vi "Main.vi"() -> ()   [LabVIEW 2018]
panel:
  out "Temp Dif  Down":dbl[unit](slide) scale=15.0..70.0
  out "Temp Dif  Up":dbl[unit](slide) scale=15.0..70.0
  out "Target Flow Evaporation Water":dbl[unit](slide)
  out "Temp Dif Down":dbl[unit]
  out "Temp Dif  Up":dbl[unit]
  out "Target Flow Evaporation Water":dbl[unit]
  out "Comp":bool
  in  "The Data are Stable\nPlease Save them!":bool
  in  "element 12":string
  in  "element 13":string
  in  "element 14":string
  in  "FileName":string="data"
  out "Temp Eva Water IN":dbl[unit]
  out "Run Program":bool
  out "Voltage Level FlowMeter Air ZeroFlow":dbl
  out "Voltage Level FlowMeter.Pre.EVA Ziro Flow Water":dbl
  out "Voltage Level FlowMeter.EVA ZiroFlow Water":dbl
  out "Humidity 3rd":dbl
  out "Humidity Evaporator IN":dbl
  out "Humidity Evaporator OUT":dbl
  out "Temp 3rd Air":dbl[unit]
  out "Temp Evaporator Air IN":dbl[unit]
  out "Temp Evaporator Air OUT":dbl[unit]
  out "Voltage Level Flowmeter Air":dbl
  out "Voltage Level Flowmeter.Pre Eva Water":dbl
  out "Voltage Level Flowmeter.EVA Water":dbl
  out "Temp water  Series 2":dbl[unit]
  out "Temp Pre Eva  Water OUT":dbl[unit]
  out "Temp Pre Eva water IN":dbl[unit]
  out "Temp Evaporator Water IN":dbl[unit]
  out "Temp Evaporator Water  Out":dbl[unit]
  in  "Calibration":bool
  out "SHT/H":dbl[](array[numeric])
  out "SHT/T":dbl[unit][](array[numeric])
  out "EEP":dbl[](array[numeric])
  out "MPX":dbl[](array[numeric])
  out "DS18b20":dbl[unit][](array[numeric])
  out "Flow Evaporation Water Detected by sensor":dbl[unit](slide)
  out "Flow Evaporation Water Detected by sensor":dbl[unit]
  out "S1 is greater Than S2\nThat is Wrong":bool
  out "T_WD":dbl[unit]
  out "Temp Eva Water Out":dbl[unit](slide) scale=15.0..70.0
  out "Temp Eva Air OUT":dbl[unit](slide) scale=15.0..70.0
  out "LMTD":dbl[unit](knob) scale=0.0..5.0
  out "LMTD":dbl[unit]
  out "Pre Evaporation Water Flow Detected by sensor":dbl[unit]
  out "Pre Evaporation Water Flow Detected by sensor":dbl[unit](slide)
  out "Temp Eva Air IN":dbl[unit](slide) scale=15.0..70.0
  out "Humidity Evaporator Air Input":dbl(knob) scale=30.0..100.0
  out "Temp Eva Water IN":dbl[unit](slide) scale=15.0..70.0
  out "MFRHA\nMass Flow Rate of Humid Air \nof Input(Kg/s)":dbl[unit]
  out "Added Vapor (kg/s)":dbl[unit]
  out "Total Transferd Energy of Air":dbl[unit]
  out "Total Transferd Energy of Air":dbl[unit](knob)
  out "Mass Flow Rate of Coil Water":dbl[unit]
  out "Mass Flow Rate of Coil Water":dbl[unit](slide)
  out "Temp Eva Air IN":dbl[unit]
  out "Humidity Evaporator Air Input":dbl
  in  "Gas Presure":dbl[unit]=80000.0 min=80000.0 max=120000.0
  out "Humidity Evaporator Air OUT\nRH Heat Exchanger Quality":dbl
  out "Humidity Evaporator Air OUT\nRH Heat Exchanger Quality":dbl(knob) scale=30.0..100.0
  out "Temp Eva Air OUT":dbl[unit]
  in  "stop":bool
  in  "Run Program":bool
  out "PortName":string
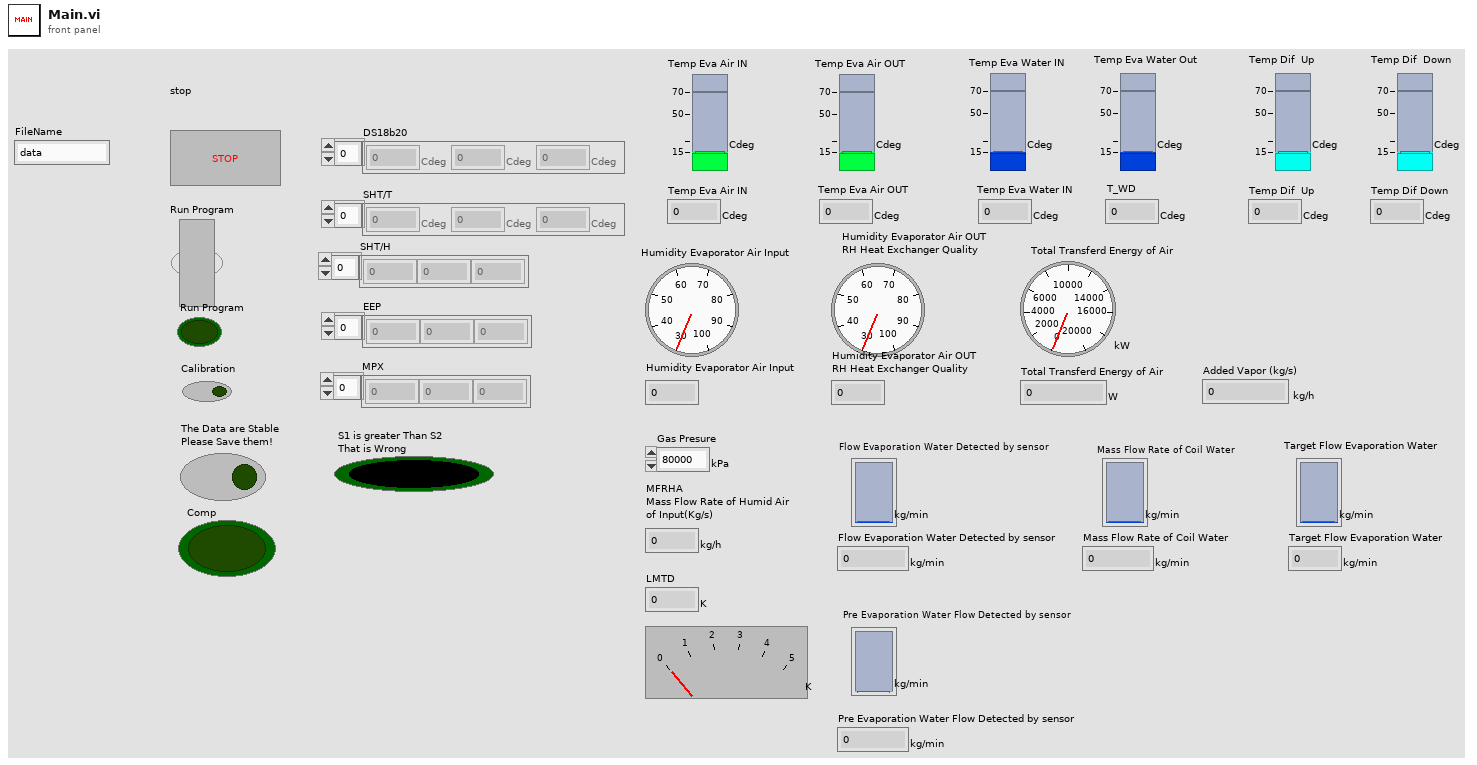
[diagram p1: front panel]
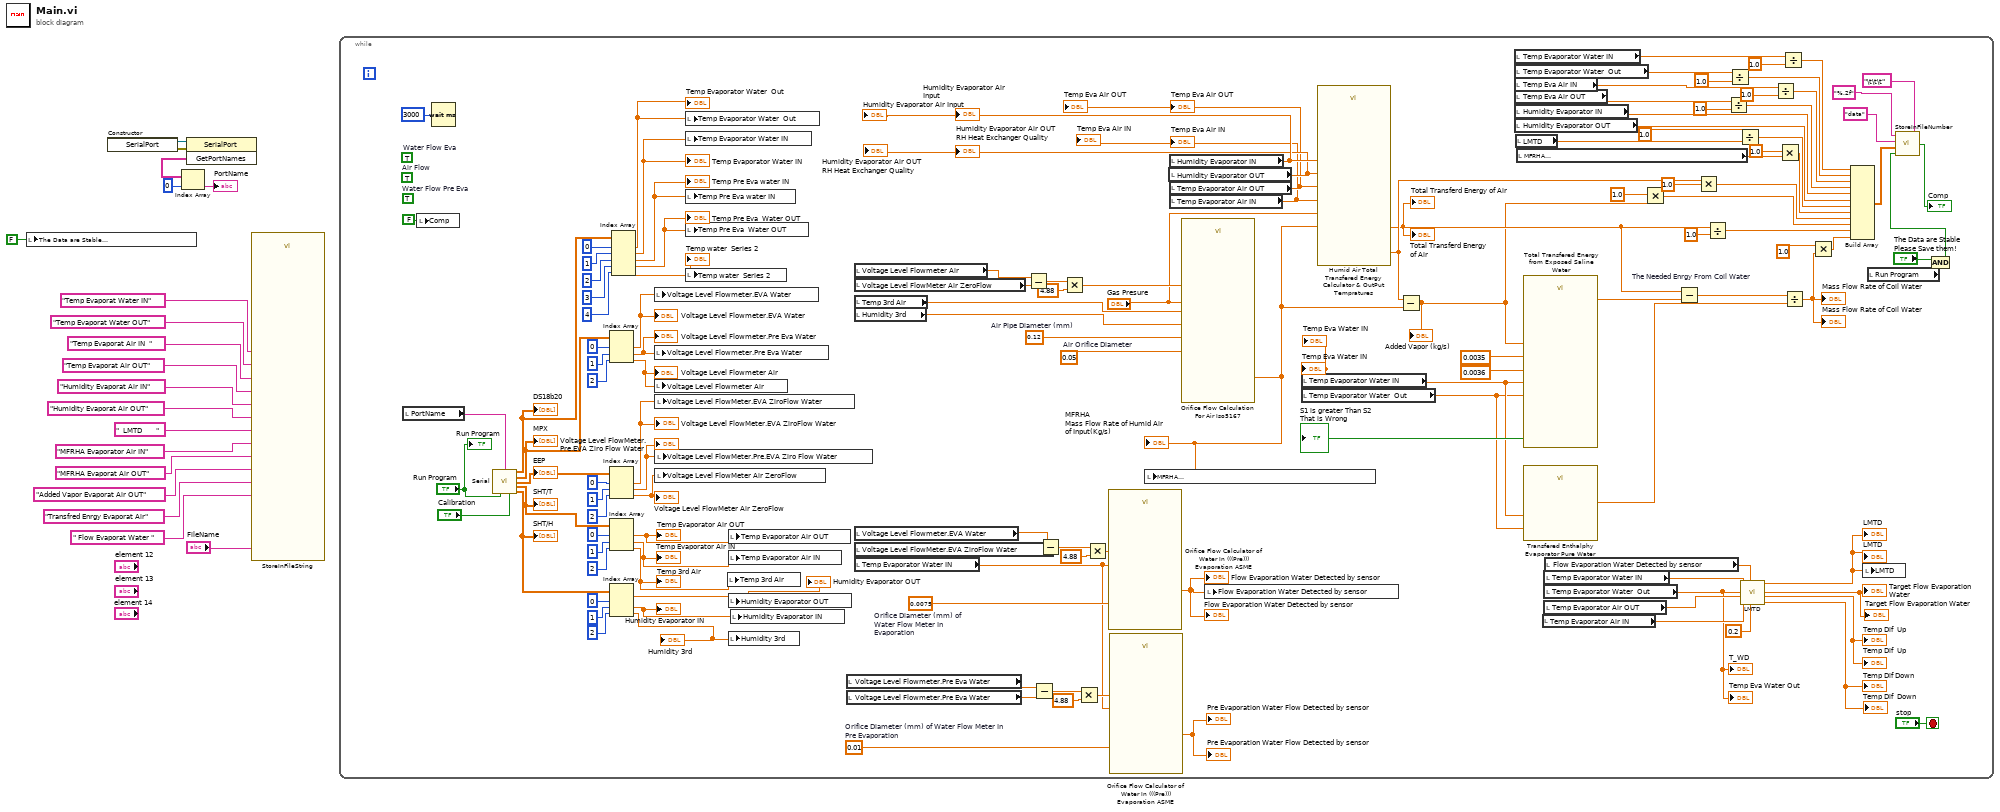
[diagram p0: block diagram]
diagram:
  n1 = local write "The Data are Stable\nPlease Save them!"(FALSE ("The Data are Stable\nPlease Save them!")) -> ()
  n2 = constructor class="SerialPort"() -> (reference out=w17:refnum<k24>, error out=w18:errorcluster)  [unwired: 3 in, 1 out]
  n3 = invoke class="SerialPort" method="GetPortNames"(reference=w17, error in=w18) -> ("GetPortNames"=w16:string[])  [unwired: 1 in, 2 out]
  n4 = Index Array(array=w16, index=0) -> (element=→"PortName":string)
  n5 = call "StoreInFileString.vi"("element0"="Temp Evaporat Water IN", "element 5"="Humidity Evaporat Air OUT", "element 6"="  LMTD       ", "element 7"="MFRHA Evaporator Air IN", "element 8"="MFRHA Evaporat Air OUT" ("element 9"), "element1"="Temp Evaporat Water OUT", "element 9"="Added Vapor Evaporat Air OUT" ("element 8"), "element 2"="Temp Evaporat Air IN  ", "element 10"="Transfred Enrgy Evaporat Air" ("element 11"), "element 3"="Temp Evaporat Air OUT", "element 11"=" Flow Evaporat Water " ("element 10"), "element 4"="Humidity Evaporat Air IN", "FileName"="FileName") -> ()  [unwired: 3 in]
  n6 = while {
    stop <- "stop" stop-if-true
    w138 = dbl[unit] 0.0075  # Orifice Diameter (mm) of Water Flow Meter In Evaporation
    w150 = dbl[unit] 0.12  # Air Pipe Diameter (mm)
    w97 = dbl[unit] 0.05  # Air Orifice Diameter
    w142 = dbl[unit] 0.01  # Orifice Diameter (mm) of Water Flow Meter In Pre Evaporation
    (unwired) TRUE  # Water Flow Eva
    (unwired) TRUE  # Water Flow Pre Eva
    (unwired) TRUE  # Air Flow
    n7 = local read "PortName"() -> (w79:string)
    n8 = local write "Comp"(FALSE ("Comp")) -> ()
    n9 = Wait (ms)(milliseconds to wait=u32 3000) -> ()  [unwired: 1 out]
    n10 = call "Serial.vi"("PortName"=w79, "Run"="Run Program", "Calibration"="Calibration") -> ("DS18b20"=w136:dbl[unit][], "MPX"=w130:dbl[], "EEP"=w115:dbl[], "SHT/H"=w126:dbl[unit][], "SHT/T"=w116:dbl[])  [unwired: 3 in, 5 out]
    "DS18b20" <- w136
    "MPX" <- w130
    "EEP" <- w115
    "SHT/T" <- w126
    "SHT/H" <- w116
    n11 = Index Array(array=w130, index #1=0 ("index"), index #2=1 ("index"), index #3=2 ("index")) -> (element #1=w111:dbl, element #2=w110:dbl, element #3=w100:dbl)
    "Voltage Level Flowmeter.EVA Water" <- w111
    "Voltage Level Flowmeter.Pre Eva Water" <- w110
    "Voltage Level Flowmeter Air" <- w100
    n12 = Index Array(array=w115, index #1=0 ("index"), index #2=1 ("index"), index #3=2 ("index")) -> (element #1=w109:dbl, element #2=w108:dbl, element #3=w107:dbl)
    "Voltage Level FlowMeter.EVA ZiroFlow Water" <- w109
    "Voltage Level FlowMeter.Pre.EVA Ziro Flow Water" <- w108
    "Voltage Level FlowMeter Air ZeroFlow" <- w107
    n13 = Index Array(array=w126, index #1=0 ("index"), index #2=1 ("index"), index #3=2 ("index")) -> (element #1=w105:dbl[unit], element #2=w106:dbl[unit], element #3=w104:dbl[unit])
    "Temp Evaporator Air OUT" <- w105
    "Temp Evaporator Air IN" <- w106
    "Temp 3rd Air" <- w104
    n14 = Index Array(array=w116, index #1=0 ("index"), index #2=1 ("index"), index #3=2 ("index")) -> (element #1=w102:dbl, element #2=w85:dbl, element #3=w103:dbl)
    "Humidity Evaporator OUT" <- w102
    "Humidity Evaporator IN" <- w85
    "Humidity 3rd" <- w103
    n15 = Index Array(array=w136, index #1=0 ("index"), index #2=1 ("index"), index #3=2 ("index"), index #4=3 ("index"), index #5=4 ("index")) -> (element #1=w68:dbl[unit], element #2=w91:dbl[unit], element #3=w119:dbl[unit], element #4=w118:dbl[unit], element #5=w117:dbl[unit])
    "Temp Evaporator Water  Out" <- w68
    "Temp Evaporator Water IN" <- w91
    "Temp Pre Eva water IN" <- w119
    "Temp Pre Eva  Water OUT" <- w118
    "Temp water  Series 2" <- w117
    n16 = local write "Voltage Level Flowmeter.EVA Water"(w111) -> ()
    n17 = local write "Voltage Level Flowmeter.Pre Eva Water"(w110) -> ()
    n18 = local write "Voltage Level Flowmeter Air"(w100) -> ()
    n19 = local write "Voltage Level FlowMeter.EVA ZiroFlow Water"(w109) -> ()
    n20 = local write "Voltage Level FlowMeter.Pre.EVA Ziro Flow Water"(w108) -> ()
    n21 = local write "Voltage Level FlowMeter Air ZeroFlow"(w107) -> ()
    n22 = local write "Temp Evaporator Water  Out"(w68) -> ()
    n23 = local write "Temp Evaporator Water IN"(w91) -> ()
    n24 = local write "Temp Pre Eva water IN"(w119) -> ()
    n25 = local write "Temp Pre Eva  Water OUT"(w118) -> ()
    n26 = local write "Temp water  Series 2"(w117) -> ()
    n27 = local write "Temp 3rd Air"(w104) -> ()
    n28 = local write "Temp Evaporator Air OUT"(w105) -> ()
    n29 = local write "Temp Evaporator Air IN"(w106) -> ()
    n30 = local write "Humidity Evaporator OUT"(w102) -> ()
    n31 = local write "Humidity 3rd"(w103) -> ()
    n32 = local write "Humidity Evaporator IN"(w85) -> ()
    n33 = local read "Voltage Level Flowmeter.Pre Eva Water"() -> (w96:dbl)
    n34 = local read "Voltage Level Flowmeter.Pre Eva Water"() -> (w95:dbl)
    n35 = local read "Voltage Level Flowmeter Air"() -> (w101:dbl)
    n36 = local read "Voltage Level FlowMeter Air ZeroFlow"() -> (w99:dbl)
    n37 = local read "Temp 3rd Air"() -> (w86:dbl[unit])
    n38 = local read "Humidity 3rd"() -> (w87:dbl)
    n39 = local read "Voltage Level Flowmeter.EVA Water"() -> (w94:dbl)
    n40 = local read "Voltage Level FlowMeter.EVA ZiroFlow Water"() -> (w93:dbl)
    n41 = local read "Temp Evaporator Water IN"() -> (w92:dbl[unit])
    n42 = Subtract(x=w101, y=w99) -> (x-y=w147:dbl)
    n43 = Subtract(x=w96, y=w95) -> (x-y=w144:dbl)
    n44 = Subtract(x=w94, y=w93) -> (x-y=w140:dbl)
    n45 = Multiply(x=w147, y=dbl[unit] 4.88) -> (x*y=w151:dbl[unit])
    n46 = Multiply(x=w144, y=dbl[unit] 4.88) -> (x*y=w143:dbl[unit])
    n47 = Multiply(x=w140, y=dbl[unit] 4.88) -> (x*y=w139:dbl[unit])
    n48 = call "Orifice Flow Calculator of Water In (((Pre))) Evaporation ASME.vi"("Water Temperature"=w92, "Delta P\n(Presure Made By Orifice)"=w139, "Orifice Diameter"=w138) -> ("Mass Flow (Orifice) (Kg/min)"=w33:dbl[unit])  [unwired: 1 in, 2 out]
    "Flow Evaporation Water Detected by sensor" <- w33
    "Flow Evaporation Water Detected by sensor" <- w33
    n49 = call "Orifice Flow Calculator of Water In (((Pre))) Evaporation ASME.vi"("Water Temperature"=w92, "Delta P\n(Presure Made By Orifice)"=w143, "Orifice Diameter"=w142) -> ("Mass Flow (Orifice) (Kg/min)"=→"Pre Evaporation Water Flow Detected by sensor" →"Pre Evaporation Water Flow Detected by sensor":dbl[unit])  [unwired: 1 in, 2 out]
    n50 = local read "Humidity Evaporator OUT"() -> (w83:dbl)
    "Humidity Evaporator Air OUT\nRH Heat Exchanger Quality" <- w83
    "Humidity Evaporator Air OUT\nRH Heat Exchanger Quality" <- w83
    n51 = local read "Humidity Evaporator IN"() -> (w84:dbl)
    "Humidity Evaporator Air Input" <- w84
    "Humidity Evaporator Air Input" <- w84
    n52 = local read "Temp Evaporator Air OUT"() -> (w81:dbl[unit])
    "Temp Eva Air OUT" <- w81
    "Temp Eva Air OUT" <- w81
    n53 = local read "Temp Evaporator Air IN"() -> (w80:dbl[unit])
    "Temp Eva Air IN" <- w80
    "Temp Eva Air IN" <- w80
    n54 = call "Orifice Flow Calculation For Air Iso5167.vi"("RH"=w87, "Orifice Diameter"=w97, "Gas Temperature"=w86, "P1\n(Presure After Fan &\n before Orifice)"="Gas Presure", "Pipe Diameter (mm)"=w150, "Delta P\n(Presure Made By Orifice)"=w151) -> ("Mass Flow (Orifice) (Kg/h)"=w47:dbl[unit])  [unwired: 2 out]
    "MFRHA\nMass Flow Rate of Humid Air \nof Input(Kg/s)" <- w47
    n55 = local write "MFRHA\nMass Flow Rate of Humid Air \nof Input(Kg/s)"(w47) -> ()
    n56 = local write "Flow Evaporation Water Detected by sensor"(w33) -> ()
    n57 = local read "Temp Evaporator Water IN"() -> (w22:dbl[unit])
    "Temp Eva Water IN" <- w22
    "Temp Eva Water IN" <- w22
    n58 = local read "Temp Evaporator Water  Out"() -> (w21:dbl[unit])
    n59 = call "Humid Air Total Transfered Energy Calculator & OutPut Tempratures.vi"("MFRHA\nMass Flow Rate of Humid Air (Kg/s)"=w47, "Gas Presure"="Gas Presure", "T_AU"=w81, "Tceg"=w80, "RH Heat Exchanger Quality"=w83, "RH"=w84) -> ("Mass Flow Rate of Humid Air of Out Put"=w66:dbl[unit], "ToTal Transferd Energy of Air"=w64:dbl[unit])
    "Total Transferd Energy of Air" <- w64
    "Total Transferd Energy of Air" <- w64
    n60 = Subtract(x=w66, y=w47) -> (x-y=w26:dbl[unit])
    "Added Vapor (kg/s)" <- w26
    n61 = local read "Temp Evaporator Water IN"() -> (w76:dbl[unit])
    n62 = local read "Temp Evaporator Water  Out"() -> (w71:dbl[unit])
    n63 = local read "Temp Eva Air IN"() -> (w70:dbl[unit])
    n64 = local read "Temp Eva Air OUT"() -> (w69:dbl[unit])
    n65 = local read "Humidity Evaporator IN"() -> (w51:dbl)
    n66 = local read "Humidity Evaporator OUT"() -> (w50:dbl)
    n67 = local read "LMTD"() -> (w41:dbl[unit])
    n68 = local read "MFRHA\nMass Flow Rate of Humid Air \nof Input(Kg/s)"() -> (w57:dbl[unit])
    n69 = call "Total Transfered Energy from Exposed Saline Water.vi"("Adde Vapor"=w26, "Salinity Evaporator Water OUT"=0.0036 ("Salinity of Output Exposed\n Saline Water"), "Salinity Evaporator Water IN"=0.0035 ("Salinity of Input Exposed \nSaline Water"), "Temp Evap Water OUT"=w21, "Temp Evap Water IN"=w22) -> ("S1 is greater Than S2\nThat is Wrong"=→"S1 is greater Than S2\nThat is Wrong":bool, "Total Transfered Energy from Exposed Saline Water"=w23:dbl[unit])  [unwired: 2 out]
    n70 = call "Transfered Enthalphy Evaporator Pure Water.vi"("Temp Evap Water OUT"=w21, "Temp Evap Water IN"=w22) -> ("Transfered Enthalphy Evaporator (Pure) Water"=w20:dbl[unit])
    n71 = local read "Temp Evaporator Air IN"() -> (w88:dbl[unit])
    n72 = local read "Temp Evaporator Water IN"() -> (w90:dbl[unit])
    n73 = local read "Temp Evaporator Water  Out"() -> (w82:dbl[unit])
    "Temp Eva Water Out" <- w82
    "T_WD" <- w82
    n74 = local read "Temp Evaporator Air OUT"() -> (w89:dbl[unit])
    n75 = local read "Flow Evaporation Water Detected by sensor"() -> (w32:dbl[unit])
    n76 = Multiply(x=dbl[unit] 1.0, y=w26) -> (x*y=w37:dbl)
    n77 = Subtract "The Needed Enrgy From Coil Water"(x=w64, y=w23) -> (x-y=w148:dbl[unit])
    n78 = Multiply(x=w66, y=dbl[unit] 1.0 ("x")) -> (x*y=w38:dbl)
    n79 = Divide(x=w64, y=dbl[unit] 1.0) -> (x/y=w36:dbl)
    n80 = Divide(x=w69, y=dbl[unit] 1.0) -> (x/y=w52:dbl)
    n81 = Divide(x=w71, y=dbl[unit] 1.0) -> (x/y=w54:dbl)
    n82 = Divide(x=dbl[unit] 1.0 ("y"), y=w41) -> (x/y=w40:dbl)
    n83 = call "LMTD.vi"("K"=0.2, "Current Flow"=w32, "Water Down/out Temp"=w88, "Air Down/In Temp"=w89, "Air  UP/Out Temp"=w82, "Water Up/In Temp"=w90) -> ("Temp Dif Down"=→"Temp Dif Down" →"Temp Dif  Down":dbl[unit], "Temp Dif  Up"=→"Temp Dif  Up" →"Temp Dif  Up":dbl[unit], "LMTD"=w34:dbl[unit], "Target Water Flow"=→"Target Flow Evaporation Water" →"Target Flow Evaporation Water":dbl[unit])  [unwired: 1 out]
    "LMTD" <- w34
    "LMTD" <- w34
    n84 = Divide(x=w70, y=dbl[unit] 1.0) -> (x/y=w53:dbl)
    n85 = Multiply(x=dbl[unit] 1.0, y=w57) -> (x*y=w39:dbl)
    n86 = Divide(x=w76, y=dbl[unit] 1.0) -> (x/y=w59:dbl)
    n87 = Divide(x=w148, y=w20) -> (x/y=w49:dbl[unit])
    "Mass Flow Rate of Coil Water" <- w49
    "Mass Flow Rate of Coil Water" <- w49
    n88 = Multiply(x=dbl[unit] 1.0, y=w49) -> (x*y=w35:dbl)
    n89 = Build Array(w59, w54, w53, w52, w51, w50, w40, w39, w38, w37, w36, w35) -> (w58:dbl[])
    n90 = local write "LMTD"(w34) -> ()
    n91 = local read "Run Program"() -> (w43:bool)
    n92 = And(x="The Data are Stable\nPlease Save them!", y=w43) -> (x .and. y?=w44:bool)
    n93 = call "StoreInFileNumber.vi"("delimiter"="\t\t\t", "Enable"=w44, "Data"=w58, "FileName"="data", "format"="%.2f") -> ("Comp"=→"Comp":bool)  [unwired: 1 in]
    "Run Program" <- "Run Program"
  }
